vi "FancyPID.vi"(6 "Reset PID":bool, 10 "Process Variable":dbl, 11 "Setpoint":dbl) -> (3 "Output":dbl)   [LabVIEW 2016]
uses:
  <vilib>/addons/control/pid/pid.llb/PID (DBL).vi
  <vilib>/addons/control/pid/NI_PID_pid.lvlib
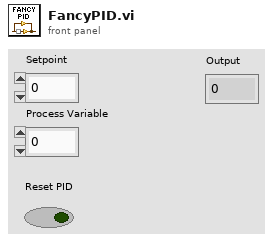
[diagram p1: front panel]
types:
  T1 = cluster{"proportional gain (Kc)":dbl, "integral time (Ti, min)":dbl, "derivative time (Td, min)":dbl}
  T2 = cluster{"proportional gain (Kc)":dbl, "f":dbl, "derivative time (Td, min)":dbl}
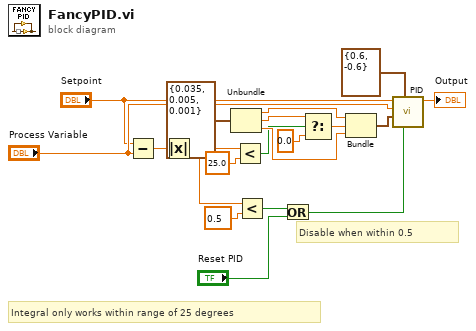
[diagram p0: block diagram]
diagram:
  # "Disable when within 0.5"
  # "Integral only works within range of 25 degrees"
  n1 = Subtract(x="Setpoint", y="Process Variable") -> (x-y=w17:dbl)
  n2 = Absolute Value(x=w17) -> (abs(x)=w8:dbl)
  n3 = Unbundle(T1 {"proportional gain (Kc)"=0.035, "integral time (Ti, min)"=0.005, "derivative time (Td, min)"=0.001} ("Angle Gains")) -> ("proportional gain (Kc)"=w16:dbl, "integral time (Ti, min)"=w14:dbl, "derivative time (Td, min)"=w15:dbl)
  n4 = Less?(x=w8, y=25.0) -> (x < y?=w13:bool)
  n5 = Less?(x=w8, y=0.5) -> (x < y?=w5:bool)
  n6 = Or(x=w5, y="Reset PID") -> (x .or. y?=w4:bool)
  n7 = Select(t=w14, s=w13, f=0.0) -> (s? t:f=w11:dbl)
  n8 = Bundle("proportional gain (Kc)"=w16, "f"=w11, "derivative time (Td, min)"=w15) -> (w10:T2)  [unwired: 1 in]
  n9 = call-poly <vilib>:"PID.vi"("reinitialize? (F)"=w4, "output range"=cluster{"output high":dbl, "output low":dbl} {"output high"=0.6, "output low"=-0.6}, "PID gains"=w10, "process variable"="Process Variable", "setpoint"="Setpoint") -> ("output"=→"Output":dbl)  [unwired: 5 in, 1 out]
